vi "JSONRPC-GetNextValue.vi"(7 "unquote strings (false)":bool, 11 "input string":string) -> (2 "after":string, 3 "next":string)   [LabVIEW 2019]
doc: "Search for the next array element in <b>input string</b>."
uses:
  <vilib>/regexp/Match Regular Expression.xnode
panel:
  # "GetNextValue"
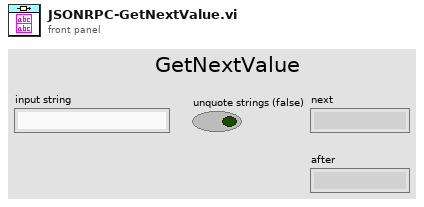
[diagram p1: front panel]
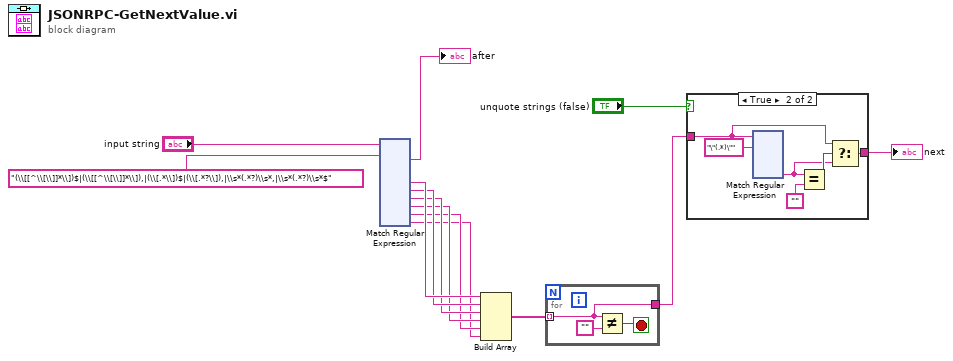
[diagram p0: block diagram]
diagram:
  n1 = xnode "Match Regular Expression"("input string"="input string", "regular expression"="(\\[[^\\[\\]]*\\])$|(\\[[^\\[\\]]*\\]),|(\\[.*\\])$|(\\[.*?\\]),|\\s*(.*?)\\s*,|\\s*(.*?)\\s*$" ("input string")) -> ("after match"=→"after":string, "submatch 1"=w8:string, "submatch 2"=w7:string, "submatch 3"=w6:string, "submatch 4"=w5:string, "submatch 5"=w2:string, "submatch 6"=w1:string)  [unwired: 4 in, 4 out]
  n2 = Build Array(w8, w7, w6, w5, w2, w1) -> (w4:string[])
  n3 = for {
    tunnel: w4 -> [w15] mode=indexing
    tunnel: [w15] -> w3
    stop <- w14 stop-if-true
    n4 = Not Equal?(x=w15, y="") -> (x != y?=w14:bool)
  }
  n5 = case shown="True" "unquote strings (false)" {
    tunnel: w3 -> [w17 w18]
    tunnel: [w17 w19] -> w10
    frame False {
    }
    frame True {
      n6 = xnode "Match Regular Expression"("input string"=w18, "regular expression"="\"(.*)\"") -> ("submatch 1"=w20:string)  [unwired: 4 in, 5 out]
      n7 = Equal?(x=w20, y="") -> (x = y?=w21:bool)
      n8 = Select(t=w18, s=w21, f=w20) -> (s? t:f=w19:string)
    }
  }
  "next" <- w10
